vi "Robot Global Data.vi"() -> ()   [LabVIEW 2014]
doc: "This global VI can contain as many global variables as you need. Place a control on the panel, give it a good name. To read or write to it from a VI, drag the icon to the diagram of that VI. You can also drag from the project. Click on the node to change which global you access. You shouldn't have multiple locations writing to a global or it will cause a race-condition."
uses:
  <vilib>/Rock Robotics/WPI/Camera/WPI_CameraImageSize.ctl
  <vilib>/Rock Robotics/WPI/DriverStation/WPI_DriverStationRobotMode2.ctl
panel:
  in  "# of Totes":dbl
  in  "Ramp Location":enum16{"High", "Low"}(ring)
  in  "Lift Manual Speed":dbl
  in  "Arm Manual Speed":dbl
  in  "Arm State":enum16{"Initializing", "Running", "Manual"}(ring)
  in  "Lift State":enum16{"Initializing", "Running", "Manual"}(ring)
  in  "Robot Arm Location":enum16{"High", "Low"}(ring)
  in  "Primary Mode":enum16{"Joysticks", "Xbox"}(ring)
  out "Lift Initialized":bool
  in  "Wrist Speed":dbl
  in  "Clamp open":bool
  in  "Axis Controls Secondary":T1(array[ring])
  in  "Button controls Secondary":T2(array[ring])
  in  "Button Controls Primary":T3(array[ring])
  in  "Axis Controls Primary":T4(array[ring])
  in  "Robot Lift Location":enum16{"High", "Low"}(ring)
  in  "Drive Controls":T5
  in  "Variables":string[](array[string])
  in  "Robot Mode":T6
  in  "image size":T7=enum."320x240"
  in  "Enable Vision":bool
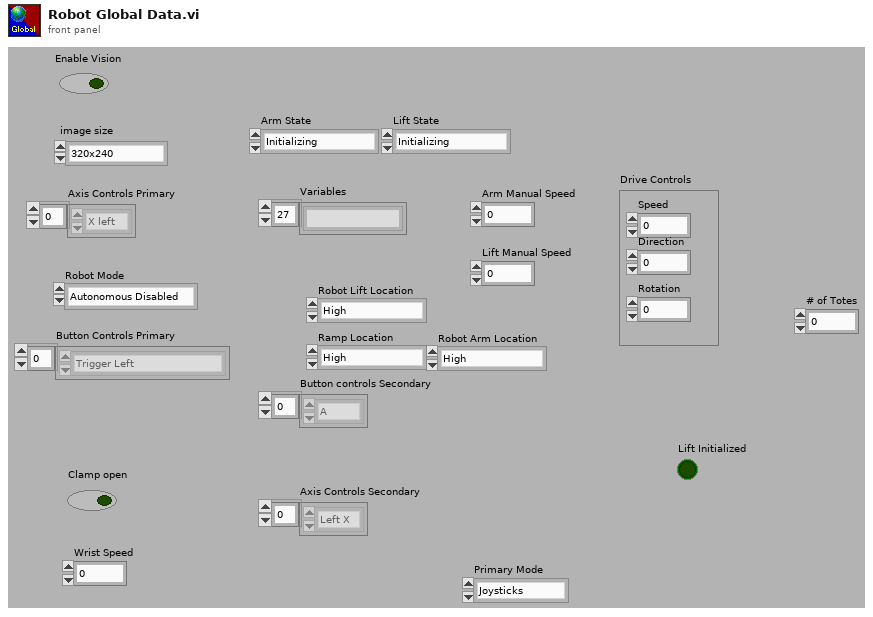
[diagram p1: front panel]
types:
  T1 = enum16{"Left X", "Left Y", "Left trigger", "R trigger", "R X", "R Y"}[]
  T2 = enum16{"A", "B", "X", "Y", "Left bumper", "Right bumper", "Back", "Start", "Left Joystick down", "Right Joystick down"}[]
  T3 = enum16{"Trigger Left", "2 Left", "3 Left", "4 Left", "5 Left", "6 Left", "7 Left", "8 Left", "9 Left", "10 Left", "11 Left", "Trigger Right", "2 Right", "3 Right", "4 Right", "5 Right", "6 Right", "7 Right", "8 Right", "9 Right", "10 Right", "11 Right"}[]
  T4 = enum16{"X left ", "Y left", "Z left", "X right", "Y right", "Z right"}[]
  T5 = cluster{"Speed":dbl, "Direction":dbl, "Rotation":dbl}
  T6 = typedef "WPI_DriverStationRobotMode2.ctl" = enum16{"Autonomous Disabled", "Autonomous Enabled", "Teleop Disabled", "Teleop Enabled", "Disconnected", "Finish", "Test Disabled", "Test Enabled", "Emergency Stopped"}
  T7 = typedef "WPI_CameraImageSize.ctl" = enum16{"640x480", "320x240", "160x120", "Custom"}
diagram:
